vi "location ini.vi"(8 "read/write":enum16{"Write", "Read"}(ring), 11 "Location In":cluster{"City":string, "State":string}) -> (3 "Location Out":cluster{"City":string, "State":string})   [LabVIEW 2015]
uses:
  Process Controller 3.0/Calibration and Function folders.ctl
  <vilib>/Utility/config.llb/Write Key (String).vi
  <vilib>/Utility/config.llb/Read Key (String).vi
  <vilib>/Utility/config.llb/NI_LVConfig.lvlib
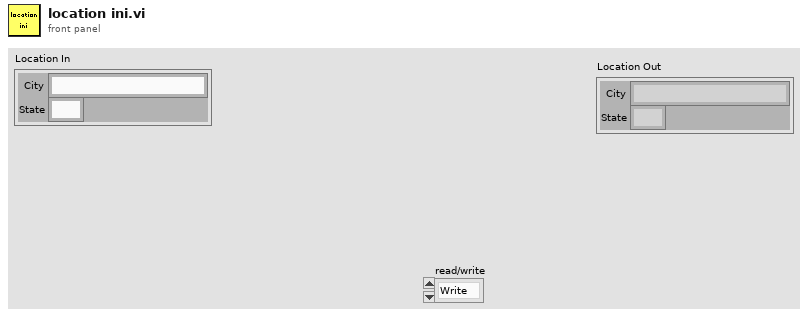
[diagram p1: front panel]
types:
  T1 = typedef "Calibration and Function folders.ctl" = enum16{"Sensors", "Functions", "Config File", "PublicAppFolder", "New ini File", "Set Config File", "Delete ini File"}
  T2 = typedef "NI_LVConfig.lvlib/Config Data RefNum.ctl" = refnum<k1>
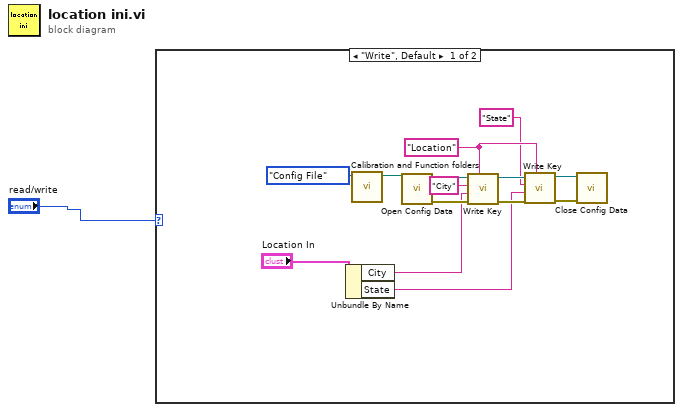
[diagram p0: block diagram]
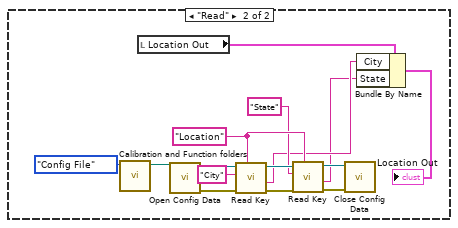
[diagram p2: hidden frame]
diagram:
  n1 = case shown="\"Write\", Default" "read/write" {
    frame "Write", Default {
      w6 = "Location" ("section")
      n2 = Unbundle By Name("Location In") -> ("City"=w9:string, "State"=w5:string)
      n3 = call "Calibration and Function folders.vi"("Folder"=Calibration_and_Function_folders."Config File") -> ("Selected Folder"=w14:path)  [unwired: 9 in, 1 out]
      n4 = call <vilib>:"Open Config Data.vi"("configuration file path"=w14) -> ("error out"=w12:errorcluster, "refnum"=w15:T2)  [unwired: 8 in, 1 out]
      n5 = call-poly <vilib>:"Write Key.vi"("section"=w6, "error in (no error)"=w12, "value"=w9, "key"="City", "refnum"=w15) -> ("error out"=w8:errorcluster, "refnum out"=w7:T2)  [unwired: 4 in, 1 out]
      n6 = call-poly <vilib>:"Write Key.vi"("section"=w6, "error in (no error)"=w8, "value"=w5, "key"="State", "refnum"=w7) -> ("error out"=w3:errorcluster, "refnum out"=w2:T2)  [unwired: 4 in, 1 out]
      n7 = call <vilib>:"Close Config Data.vi"("error in (no error)"=w3, "refnum"=w2) -> ()  [unwired: 8 in, 2 out]
    }
    frame "Read" {
      w23 = "Location" ("section")
      n8 = call "Calibration and Function folders.vi"("Folder"=Calibration_and_Function_folders."Config File") -> ("Selected Folder"=w29:path)  [unwired: 9 in, 1 out]
      n9 = local read "Location Out"() -> (w19:cluster{"City":string, "State":string})
      n10 = call <vilib>:"Open Config Data.vi"("configuration file path"=w29) -> ("error out"=w27:errorcluster, "refnum"=w30:T2)  [unwired: 8 in, 1 out]
      n11 = call-poly <vilib>:"Read Key.vi"("section"=w23, "error in (no error)"=w27, "key"="City", "refnum"=w30) -> ("error out"=w25:errorcluster, "value"=w18:string, "refnum out"=w24:T2)  [unwired: 4 in, 1 out]
      n12 = call-poly <vilib>:"Read Key.vi"("section"=w23, "error in (no error)"=w25, "key"="State", "refnum"=w24) -> ("error out"=w22:errorcluster, "value"=w17:string, "refnum out"=w21:T2)  [unwired: 4 in, 1 out]
      n13 = call <vilib>:"Close Config Data.vi"("error in (no error)"=w22, "refnum"=w21) -> ()  [unwired: 8 in, 2 out]
      n14 = Bundle By Name(cluster=w19, "City"=w18, "State"=w17) -> (→"Location Out":cluster{"City":string, "State":string})
    }
  }
